vi "ComTool_360.vi"(0 "Com":refnum<visa-resource-name>, 1 "SN":string, 2 "DevID":string, 5 "通信协议名称":string, 7 "DelayTime":u32, 9 "F0?":bool, 11 "error in":errorcluster caption="错误输入（无错误）", 12 "Debug":bool=TRUE) -> (4 "响应":string, 6 "反馈结果":bool, 8 "Data":string, 10 "CMD":string, 15 "error out":errorcluster caption="错误输出")   [LabVIEW 2013]
uses:
  <vilib>/Utility/NIReport.llb/NI_report.lvclass
  SourceCode/GlobalValue.vi
  <vilib>/Utility/error.llb/Error Cluster From Error Code.vi
  <vilib>/addons/_office/excel.llb/Excel Get Data ([str]).vi
  <vilib>/ErrorRing/Error Ring.xnode
  <vilib>/addons/_office/NI_ReportGenerationToolkit.lvlib
  <vilib>/Utility/NIReport.llb/Excel/NI_Excel.lvclass
panel:
  out "应答列表":u16(ring) items=["握手命令应答", "模拟数据清除应答", "模拟车速应答", "模拟方向盘角度应答", "模拟OFF档应答", "模拟ACC档应答", "模拟ON档应答", "模拟RUN档应答", "模拟气囊打开应答", "模拟气囊关闭应答", "模拟转向正常应答", "模拟左转应答", "模拟右转应答", "模拟转向报警应答", "模拟N档应答", "模拟R档应答", "模拟R+左转应答", "模拟R+右转应答", "模拟L档应答", "模拟S档应答", "模拟D档应答", "模拟P档应答", "模拟5档应答", "打开AVM输出应答", "关闭AVM输出应答", "获取MCU-APP版本应答", "获取MCU-BOOT版本应答", "重启应答", "获取ARM-APP版本应答", "获取ARM算法版本应答", "2D前视视角应答", "2D后视视角应答", "2D左视视角应答", "2D右视视角应答", "3D前视视角应答", "3D右前视角应答", "3D右后视角应答", "3D后视视角应答", "3D左后视角应答", "3D左前视角应答", "3D倒车视角应答", "3D自定义角度视角应答", "查询当前视图应答", "打开视频标定应答", "关闭视频标定应答", "设置车模红色应答", "设置车模白色应答", "设置车模银色应答", "设置车模灰色应答", "设置车模绿色应答", "设置车模紫色应答", "打开AVM总开关应答", "关闭AVM总开关应答", "打开前静态轨迹线应答", "关闭前静态线轨迹应答", "打开后静态轨迹线应答", "关闭后静态轨迹线应答", "打开后动态轨迹线应答", "关闭后动态轨迹线应答", "打开左右指引线应答", "关闭左右指引线应答", "打开LDW应答", "关闭LDW应答", "打开BSD应答", "关闭BSD应答", "打开DOW应答", "关闭DOW应答", "打开CTA应答", "关闭CTA应答", "设置LDW速度为0应答", "设置LDW速度为20应答", "设置LDW速度为40应答", "设置LDW速度为60应答", "设置BSD速度为0应答", "设置BSD速度为20应答", "设置BSD速度为40应答", "设置BSD速度为60应答", "设置DOW速度为0应答", "设置DOW速度为20应答", "设置DOW速度为40应答", "设置DOW速度为60应答", "设置CTA速度为0应答", "设置CTA速度为20应答", "设置CTA速度为40应答", "设置CTA速度为60应答", "获取AVM设置参数应答", "设置开启转向使能应答", "设置关闭转向使能应答", "写入主机条码应答", "读取主机条码应答", "写入设备ID应答", "读取设备ID应答", "停止测试应答", "切换2D显示应答", "切换3D显示应答", "SD卡测试应答", "MCU休眠指令应答", "ACC电压检测应答", "U盘检测应答"]
  out "读取缓存区":string
  in  "默认终止符":bool
  out "Time(ms)":u32
  out "ConfigPath":string
  out "命令":string
  out "字符串数值":bool
  out "data":string
  in  "命令列表":u16(ring) items=["握手命令", "模拟数据清除", "模拟车速", "模拟方向盘角度", "模拟OFF档", "模拟ACC档", "模拟ON档", "模拟RUN档", "模拟气囊打开", "模拟气囊关闭", "模拟转向正常", "模拟左转", "模拟右转", "模拟转向报警", "模拟N档", "模拟R档", "模拟R+左转", "模拟R+右转", "模拟L档", "模拟S档", "模拟D档", "模拟P档", "模拟5档", "打开AVM输出", "关闭AVM输出", "获取MCU-APP版本", "获取MCU-BOOT版本", "重启", "获取ARM-APP版本", "获取ARM算法版本", "2D前视视角", "2D后视视角", "2D左视视角", "2D右视视角", "3D前视视角", "3D右前视角", "3D右后视角", "3D后视视角", "3D左后视角", "3D左前视角", "3D倒车视角", "3D自定义角度视角", "查询当前视图", "打开视频标定", "关闭视频标定", "设置车模红色", "设置车模白色", "设置车模银色", "设置车模灰色", "设置车模绿色", "设置车模紫色", "打开AVM总开关", "关闭AVM总开关", "打开前静态轨迹线", "关闭前静态线轨迹", "打开后静态轨迹线", "关闭后静态轨迹线", "打开后动态轨迹线", "关闭后动态轨迹线", "打开左右指引线", "关闭左右指引线", "打开LDW", "关闭LDW", "打开BSD", "关闭BSD", "打开DOW", "关闭DOW", "打开CTA", "关闭CTA", "设置LDW速度为0", "设置LDW速度为20", "设置LDW速度为40", "设置LDW速度为60", "设置BSD速度为0", "设置BSD速度为20", "设置BSD速度为40", "设置BSD速度为60", "设置DOW速度为0", "设置DOW速度为20", "设置DOW速度为40", "设置DOW速度为60", "设置CTA速度为0", "设置CTA速度为20", "设置CTA速度为40", "设置CTA速度为60", "获取AVM设置参数", "设置开启转向使能", "设置关闭转向使能", "写入主机条码", "读取主机条码", "写入设备ID", "读取设备ID", "停止测试", "切换2D显示", "切换3D显示", "SD卡测试", "MCU休眠指令", "ACC电压检测", "U盘检测"]
  # "起始符分FF和F0两种,布尔变量兼并F0和FF两种情况"
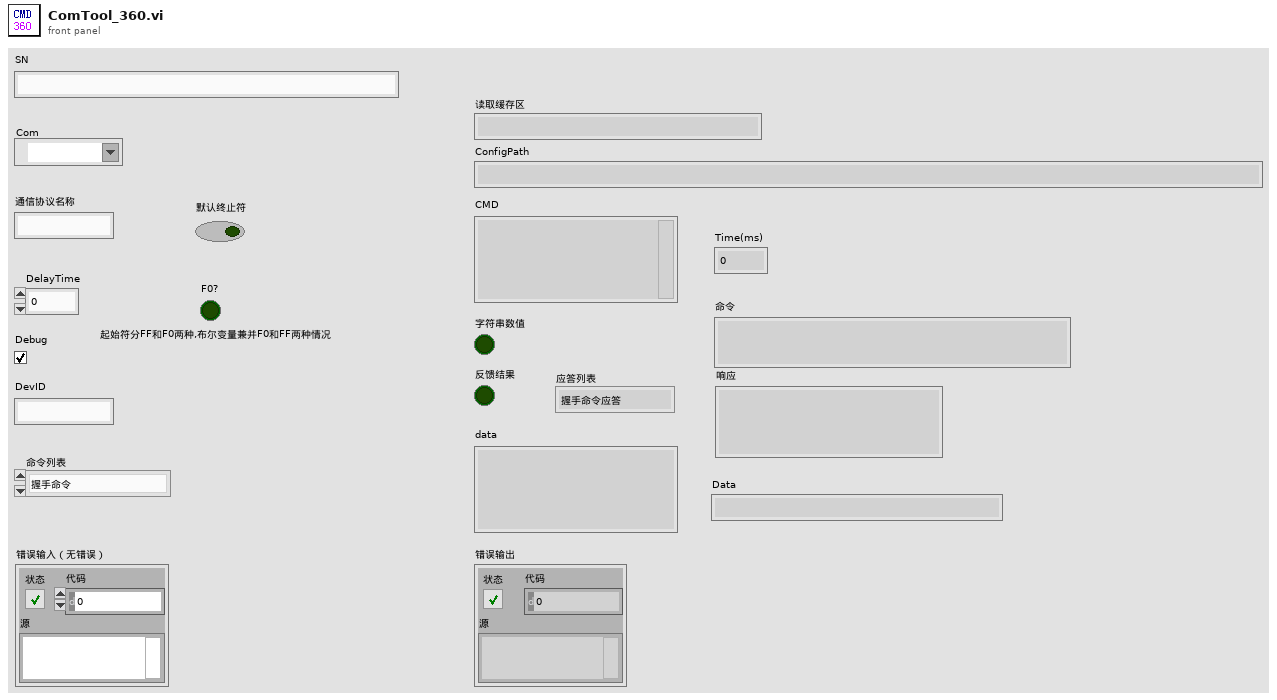
[diagram p1: front panel]
types:
  T1 = cluster{"命令码":string, "HID":string, "数据长度":string, "数据域":string}
  T2 = enum32{"invalid app kind", "Development System", "Run Time System", "Student Edition", "Embedded LabVIEW", "Evaluation", "Custom"}
  T3 = enum16{"Standard Report", "HTML", "Word", "Excel"}
  T4 = enum16{"maximized", "minimized", "normal", "no change"}
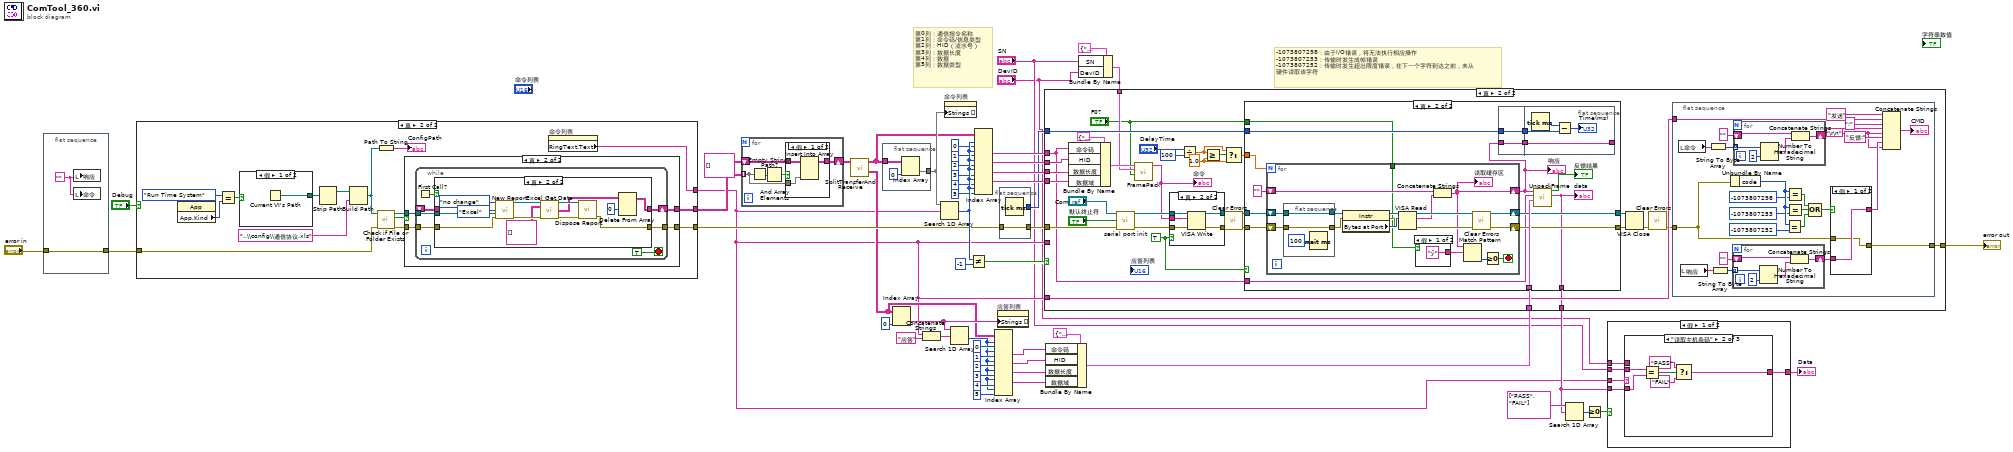
[diagram p0: block diagram]
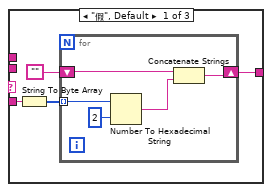
[diagram p2: hidden frame]
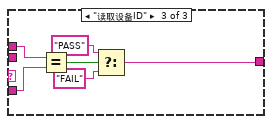
[diagram p3: hidden frame]
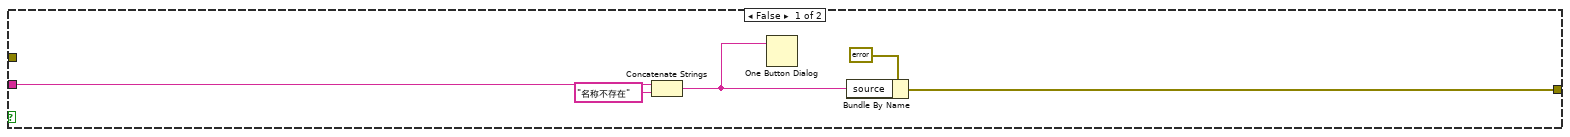
[diagram p5: hidden frame]
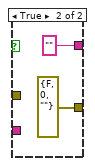
[diagram p6: hidden frame]
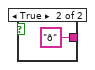
[diagram p8: hidden frame]
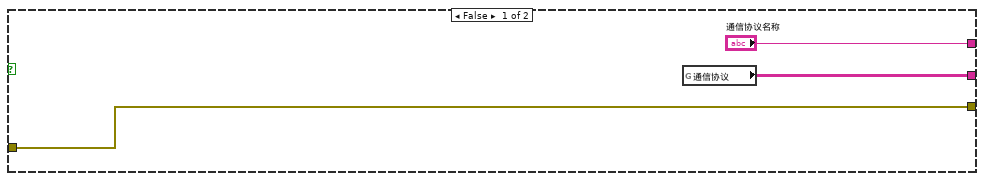
[diagram p11: hidden frame]
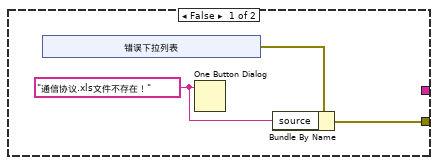
[diagram p12: hidden frame]
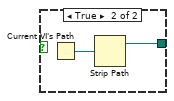
[diagram p14: hidden frame]
diagram:
  # "-1073807298：由于I/O错误，将无法执行相应操作\n-1073807253：传输时发生成帧错误\n-1073807252：传输时发生超出限度错误，在下一个字符到达之前，未从\n硬件读取该字符"
  # "第0列：通信指令名称\n第1列：命令码/信息类型\n第2列：HID（流水号）\n第3列：数据长度\n第4列：数据\n第5列：数据类型"
  n1 = flat-sequence {
    tunnel: "error in" -> [w54]
    tunnel: [w54] -> w51
    frame #0 {
      w55 = ""
      n2 = local write "响应"(w55) -> ()
      n3 = local write "命令"(w55) -> ()
    }
  }
  n4 = case shown="真" "Debug" {
    tunnel: w51 -> [w58 w65]
    tunnel: [w58 w61] -> w33
    tunnel: [w56 w60] -> w49
    tunnel: ["通信协议名称" w59] -> w3
    frame False {
      n5 = global read "GlobalValue.vi" "通信协议"() -> (w56:string[][])
    }
    frame True {
      n6 = property class="App"() -> ("App.Kind"=w72:T2)  [unwired: 2 in, 2 out]
      n7 = Equal?(x=T2."Run Time System" ("应用程序:类别"), y=w72) -> (x = y?=w71:bool)
      n8 = case shown="假" w71 {
        tunnel: [w108 w109] -> w70
        frame False {
          n9 = Current VI's Path() -> (path=w108:path)
        }
        frame True {
          n10 = Current VI's Path() -> (path=w110:path)
          n11 = Strip Path(path=w110) -> (stripped path=w109:path)  [unwired: 1 out]
        }
      }
      n12 = Strip Path(path=w70) -> (stripped path=w69:path)  [unwired: 1 out]
      n13 = Build Path(base path=w69, name or relative path="..\\config\\通信协议.xls") -> (appended path=w66:path)
      n14 = call <vilib>:"Check if File or Folder Exists.vi"("error in (no error)"=w65, "path"=w66) -> ("error out"=w63:errorcluster, "file or folder exists?"=w64:bool, "dup path"=w62:path)  [unwired: 7 in]
      n15 = Path To String(path=w66) -> (string=→"ConfigPath":string)
      n16 = case shown="真" w64 {
        tunnel: w63 -> [_ w84]
        tunnel: w62 -> [_ w85]
        tunnel: [w75 w83] -> w61
        tunnel: [_ w82] -> w60
        frame False {
          w74 = "通信协议.xls文件不存在！"
          n17 = xnode "错误下拉列表"() -> ("错误输出"=w76:errorcluster)
          n18 = One Button Dialog(message=w74) -> ()  [unwired: 1 in, 1 out]
          n19 = Bundle By Name(cluster=w76, "source"=w74) -> (w75:errorcluster)
        }
        frame True {
          n20 = while {
            shift-right: [w89] -> w82
            shift-left: _ -> [w87]
            tunnel: w85 -> [w91]
            tunnel: w84 -> [w90]
            tunnel: [w88] -> w83
            stop <- TRUE stop-if-true
            n21 = First Call?() -> (First Call?: T/F=w92:bool)
            n22 = case shown="真" w92 {
              tunnel: w91 -> [_ w105]
              tunnel: w90 -> [w93 w104]
              tunnel: [w94 w96] -> w89
              tunnel: [w93 w95] -> w88
              tunnel: w87 -> [w94 _]
              frame False {
              }
              frame True {
                n23 = call <vilib>:"New Report.vi"("window state (normal)"=T4."no change", "report type"=T3."Excel", "template (empty)"=w105, "error in (no error)"=w104) -> ("report out"=w103:refnum<class "NI_report.lvclass">, "error out"=w102:errorcluster)  [unwired: 10 in]
                n24 = call-poly <vilib>:"Excel Get Data.vi"("report in"=w103, "data type"=string[][] [], "error in (no error)"=w102) -> ("report out"=w100:refnum<class "NI_report.lvclass">, "data"=w98:string[][], "error out"=w99:errorcluster)  [unwired: 10 in]
                n25 = call-dynamic "Dispose Report.vi"("report in"=w100, "error in (no error)"=w99) -> ("error out"=w95:errorcluster)  [unwired: 13 in]
                n26 = Delete From Array(array=w98, index (row)=0) -> (array with subset deleted=w96:string[][])  [unwired: 2 in, 1 out]
              }
            }
          }
        }
      }
      n27 = property on="命令列表" class="Ring (严格)"() -> ("RingText.Text"=w59:string)  [unwired: 2 in, 2 out]
    }
  }
  n28 = for {
    shift-right: [w111] -> w46
    shift-left: string[][] [] -> [w112]
    tunnel: w49 -> [w113] mode=indexing
    n29 = Empty String/Path?(string/path=w113) -> (empty?=w115:bool[])
    n30 = And Array Elements(Boolean array=w115) -> (logical AND=w114:bool)
    n31 = case shown="假" w114 {
      tunnel: w113 -> [w118 _]
      tunnel: w112 -> [w117 w119]
      tunnel: [w116 w119] -> w111
      frame False {
        n32 = Insert Into Array(array=w117, new element=w118) -> (w116:string[][])  [unwired: 2 in]
      }
      frame True {
      }
    }
  }
  n33 = call "SplitTransferAndReceive.vi"("StrArrayIn"=w46) -> ("Receive"=w19:string[][], "Transfer"=w31:string[][])  [unwired: 8 in, 1 out]
  n34 = flat-sequence {
    tunnel: w31 -> [w122]
    tunnel: [w120] -> w48
    frame #0 {
      n35 = Index Array(array=w122, index (col)=0) -> (element=w120:string[])  [unwired: 1 in]
    }
  }
  n36 = Index Array(array=w19, index (col)=0) -> (element=w21:string[])  [unwired: 1 in]
  n37 = Concatenate Strings(w3, "应答") -> (w28:string)
  n38 = Search 1D Array(1D array=w48, element=w3) -> (index of element=w45:i32)  [unwired: 1 in]
  n39 = property on="命令列表" class="Ring (严格)"("Strings []"=w48) -> ()  [unwired: 2 in, 2 out]
  n40 = Search 1D Array(1D array=w21, element=w28) -> (index of element=w20:i32)  [unwired: 1 in]
  n41 = Not Equal?(x=w45, y=-1) -> (x != y?=w38:bool)
  n42 = Index Array(array=w31, index (row) #1=w45, index (col) #1=0, index (row) #2=w45, index (col) #2=1, index (row) #3=w45, index (col) #3=2, index (row) #4=w45, index (col) #4=3, index (row) #5=w45, index (col) #5=4, index (row) #6=w45, index (col) #6=5) -> (element #2=w37:string, element #3=w36:string, element #4=w35:string, element #5=w34:string)  [unwired: 2 out]
  n43 = Index Array(array=w19, index (row) #1=w20, index (col) #1=0, index (row) #2=w20, index (col) #2=1, index (row) #3=w20, index (col) #3=2, index (row) #4=w20, index (col) #4=3, index (row) #5=w20, index (col) #5=4, index (row) #6=w20, index (col) #6=5) -> (element #2=w17:string, element #3=w16:string, element #4=w15:string, element #5=w14:string)  [unwired: 2 out]
  n44 = property on="应答列表" class="Ring (严格)"("Strings []"=w21) -> ()  [unwired: 2 in, 2 out]
  n45 = flat-sequence {
    tunnel: w33 -> [w124]
    tunnel: [w124] -> w32
    tunnel: [w123] -> w12
    frame #0 {
      n46 = Tick Count (ms)() -> (millisecond timer value=w123:u32)
    }
  }
  n47 = Bundle By Name(cluster=T1 {"命令码"="", "HID"="", "数据长度"="", "数据域"=""} ("FramePara"), "命令码"=w17, "HID"=w16, "数据长度"=w15, "数据域"=w14) -> (w13:T1)
  n48 = Bundle By Name(cluster=cluster{"SN":string, "DevID":string} {"SN"="", "DevID"=""} ("SNorDevID"), "SN"="SN", "DevID"="DevID") -> (w10:cluster{"SN":string, "DevID":string})
  n49 = case shown="真" w38 {
    tunnel: w3 -> [w129 _]
    tunnel: [w125 w137] -> w9
    tunnel: w32 -> [_ w160]
    tunnel: w37 -> [_ w135]
    tunnel: w36 -> [_ w157]
    tunnel: w35 -> [_ w156]
    tunnel: w34 -> [_ w155]
    tunnel: w13 -> [_ w142]
    tunnel: w12 -> [_ w141]
    tunnel: w3 -> [_ w138]
    tunnel: w10 -> [_ w136]
    tunnel: [_ w133] -> w7
    frame False {
      n50 = Concatenate Strings(w129, "名称不存在" ("字符串")) -> (w127:string)
      n51 = One Button Dialog(message=w127) -> ()  [unwired: 1 in, 1 out]
      n52 = Bundle By Name(cluster=errorcluster {"status"=FALSE, "code"=0, "source"=""} ("错误常量"), "source"=w127) -> (w125:errorcluster)
    }
    frame True {
      w147 = 1.0
      w154 = TRUE
      n53 = Bundle By Name(cluster=T1 {"命令码"="", "HID"="", "数据长度"="", "数据域"=""} ("FramePara"), "命令码"=w135, "HID"=w157, "数据长度"=w156, "数据域"=w155) -> (w158:T1)
      n54 = call "serial port init.vi"("错误输入（无错误）"=w160, "海马(1)"="默认终止符", "VISA引用句柄输入"="Com") -> ("错误输出"=w144:errorcluster, "VISA引用句柄输出"=w145:refnum<visa-resource-name>)  [unwired: 7 in]
      n55 = call "FramePack.vi"("F0?"="F0?", "SNorDevID"=w136, "FramePara"=w158) -> ("CMD"=w143:string)  [unwired: 1 in, 2 out]
      "命令" <- w143
      n56 = case shown="真" w154 {
        tunnel: w145 -> [w248 w253]
        tunnel: w144 -> [w247 w252]
        tunnel: [w248 w251] -> w153
        tunnel: [w247 w250] -> w152
        tunnel: w143 -> [_ w249]
        frame False {
        }
        frame True {
          n57 = VISA Write(VISA resource name=w253, write buffer=w249, error in (no error)=w252) -> (VISA resource name out=w251:refnum<visa-resource-name>, error out=w250:errorcluster)  [unwired: 1 out]
        }
      }
      n58 = Divide(x="DelayTime", y=u32 100) -> (x/y=w148:dbl)
      n59 = Greater Or Equal?(x=w148, y=w147) -> (x >= y?=w149:bool)
      n60 = Select(t=w148, s=w149, f=w147) -> (s? t:f=w146:dbl)
      n61 = call <vilib>:"Clear Errors.vi"("error in (no error)"=w152) -> ("error out"=w132:errorcluster)  [unwired: 6 in]
      n62 = case shown="真" w154 {
        tunnel: w153 -> [w203 w217]
        tunnel: w132 -> [w202 w216]
        tunnel: w146 -> [_ w218]
        tunnel: w142 -> [_ w214]
        tunnel: w141 -> [_ w213]
        tunnel: [w203 w210] -> w139
        tunnel: [w202 w209] -> w140
        tunnel: w135 -> [_ w208]
        tunnel: [_ w205] -> w133
        tunnel: "F0?" -> [_ w204]
        frame False {
        }
        frame True {
          n63 = for {
            N: w218 -> [_]
            shift-right: [w230] -> w212
            shift-left: "" -> [w232]
            shift-right: [w234] -> w210
            shift-left: w217 -> [w241]
            shift-right: [w226] -> w209
            shift-left: w216 -> [w240]
            tunnel: w204 -> [w225]
            stop <- w228 stop-if-true
            n64 = flat-sequence {
              tunnel: w241 -> [w246]
              tunnel: w240 -> [w245]
              tunnel: [w246] -> w239
              tunnel: [w245] -> w238
              frame #0 {
                n65 = Wait (ms)(milliseconds to wait=u32 100 ("等待时间（毫秒）")) -> ()  [unwired: 1 out]
              }
            }
            n66 = property class="Instr"(reference=w239, error in=w238) -> (reference out=w236:refnum<visa-resource-name>, error out=w235:errorcluster, "Bytes at Port"=w237:u32)
            n67 = VISA Read(VISA resource name=w236, byte count=w237, error in (no error)=w235) -> (VISA resource name out=w234:refnum<visa-resource-name>, read buffer=w231:string, error out=w233:errorcluster)  [unwired: 1 out]
            n68 = case shown="假" w225 {
              tunnel: ["ÿ" "ð"] -> w227
              frame False {
              }
              frame True {
              }
            }
            n69 = Concatenate Strings(w232, w231) -> (w230:string)
            "读取缓存区" <- w230
            n70 = Match Pattern(string=w230, regular expression=w227) -> (offset past match=w229:i32)  [unwired: 1 in, 3 out]
            n71 = call <vilib>:"Clear Errors.vi"("error in (no error)"=w233) -> ("error out"=w226:errorcluster)  [unwired: 6 in]
            n72 = Greater Or Equal To 0?(x=w229) -> (x >= 0?=w228:bool)
          }
          "响应" <- w212
          n73 = flat-sequence {
            tunnel: w212 -> [w219]
            tunnel: w213 -> [w220]
            tunnel: [w220] -> w207
            tunnel: [w219] -> w206
            tunnel: w207 -> [w223]
            tunnel: w206 -> [w221]
            tunnel: [w221] -> _
            frame #0 {
            }
            frame #1 {
              n74 = Tick Count (ms)() -> (millisecond timer value=w224:u32)
              n75 = Subtract(x=w224, y=w223) -> (x-y=→"Time(ms)":u32)
            }
          }
          n76 = call "UnpackFrame.vi"("FramePara"=w214, "原指令码"=w208, "StrIn"=w212) -> ("data"=w205:string, "反馈结果"=→"反馈结果":bool)  [unwired: 6 in, 1 out]
          "data" <- w205
        }
      }
      n77 = VISA Close(VISA resource name=w139, error in (no error)=w140) -> (error out=w134:errorcluster)
      n78 = call <vilib>:"Clear Errors.vi"("error in (no error)"=w134) -> ("error out"=w131:errorcluster)  [unwired: 6 in]
      n79 = flat-sequence {
        tunnel: w131 -> [w174]
        tunnel: w138 -> [w179]
        tunnel: [w171] -> w137
        frame #0 {
          w172 = "\r\n"
          n80 = local read "命令"() -> (w168:string)
          n81 = local read "响应"() -> (w164:string)
          n82 = String To Byte Array(string=w168) -> (unsigned byte array=w169:u8[])
          n83 = String To Byte Array(string=w164) -> (unsigned byte array=w166:u8[])
          n84 = Unbundle By Name(w174) -> ("code"=w186:i32)
          n85 = for {
            tunnel: w166 -> [w192] mode=indexing
            shift-right: [w190] -> w163
            shift-left: "" -> [w188]
            n86 = Number To Hexadecimal String(1:2, 2:w192) -> (0:w189:string)
            n87 = Concatenate Strings(w188, w189) -> (w190:string)
          }
          n88 = for {
            tunnel: w169 -> [w197] mode=indexing
            shift-right: [w195] -> w167
            shift-left: "" -> [w193]
            n89 = Number To Hexadecimal String(1:2, 2:w197) -> (0:w194:string)
            n90 = Concatenate Strings(w193, w194) -> (w195:string)
          }
          n91 = Equal?(x=w186, y=-1073807252) -> (x = y?=w180:bool)
          n92 = Equal?(x=w186, y=-1073807298) -> (x = y?=w182:bool)
          n93 = Equal?(x=w186, y=-1073807253) -> (x = y?=w181:bool)
          n94 = Compound Arithmetic op=OR(w182, w181, w180) -> (w175:bool)
          n95 = case shown="假" w175 {
            tunnel: w174 -> [w198 _]
            tunnel: [w199 ""] -> w173
            tunnel: w163 -> [w199 _]
            tunnel: [w198 errorcluster {"status"=FALSE, "code"=0, "source"=""} ("错误常量")] -> w171
            frame False {
            }
            frame True {
            }
          }
          n96 = Concatenate Strings("发送", w179, ":", w167, w172, "反馈:", w173, w172) -> (→"CMD":string)
        }
      }
    }
  }
  "error out" <- w9
  n97 = Search 1D Array(1D array=string[] ["PASS", "FAIL"], element=w7) -> (index of element=w6:i32)  [unwired: 1 in]
  n98 = Greater Or Equal To 0?(x=w6) -> (x >= 0?=w5:bool)
  n99 = case shown="假" w5 {
    tunnel: w7 -> [w258 w280]
    tunnel: [w257 w280] -> w4
    tunnel: w3 -> [w256 _]
    tunnel: "SN" -> [w255 _]
    tunnel: "DevID" -> [w254 _]
    frame False {
      n100 = case shown="\"读取主机条码\"" w256 {
        tunnel: w258 -> [w260 w272 w279]
        tunnel: [w259 w268 w275] -> w257
        tunnel: w255 -> [_ w273 _]
        tunnel: w254 -> [_ _ w274]
        frame "假", Default {
          n101 = String To Byte Array(string=w260) -> (unsigned byte array=w262:u8[])
          n102 = for {
            tunnel: w262 -> [w267] mode=indexing
            shift-right: [w263] -> w259
            shift-left: "" -> [w265]
            n103 = Number To Hexadecimal String(1:i16 2 ("宽度(-)"), 2:w267) -> (0:w264:string)
            n104 = Concatenate Strings(w265, w264) -> (w263:string)
          }
        }
        frame "读取主机条码" {
          n105 = Equal?(x=w273, y=w272) -> (x = y?=w271:bool)
          n106 = Select(t="PASS", s=w271, f="FAIL") -> (s? t:f=w268:string)
        }
        frame "读取设备ID" {
          n107 = Equal?(x=w274, y=w279) -> (x = y?=w278:bool)
          n108 = Select(t="PASS", s=w278, f="FAIL") -> (s? t:f=w275:string)
        }
      }
    }
    frame True {
    }
  }
  "Data" <- w4
